vi "BLACK BOX FINDER.vi"() -> ()   [LabVIEW 2015]
uses:
  <vilib>/userdefined/High Color/IMAQdx.ctl
  <vilib>/vision/driver/NI_Vision_Acquisition_Software.lvlib
  <resource>/objmgr/imaqdx.rc
panel:
  out "Objects (real-world) (Object Tracking 1)":T1(array[cluster])
  out "Video Modes":string
  in  "Video Mode":dbl min=0.0 max=5.0 step=1.0
  in  "Camera":T2
  out "Y Resoloution":i32
  out "X Resoloution":i32
  in  "Stop 2":bool
  out "Image":T3(plugin-control)
  out "Image 2":T3(plugin-control)
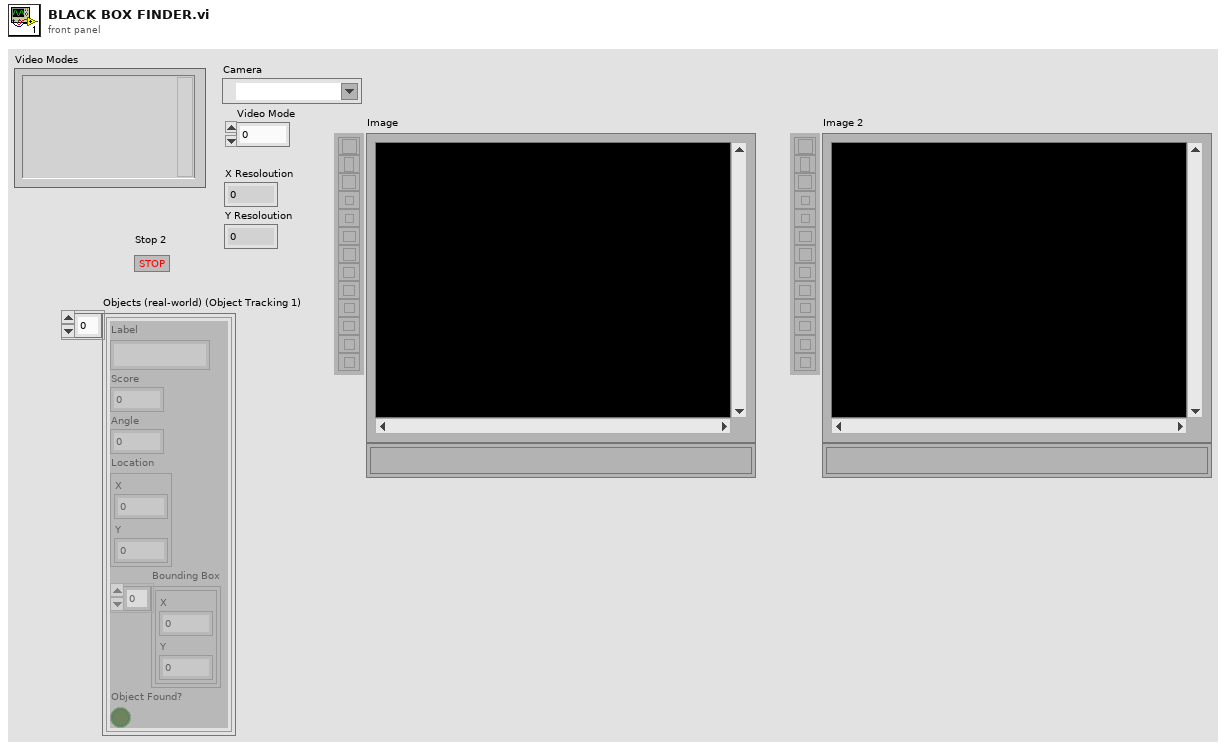
[diagram p1: front panel]
types:
  T1 = cluster{"Label":string, "Score":i32, "Angle":dbl, "Location":cluster{"X":dbl, "Y":dbl}, "Bounding Box":cluster{"X":dbl, "Y":dbl}[], "Object Found?":bool}[]
  T2 = typedef "IMAQdx.ctl" = refnum<k21>
  T3 = typedef "IMAQ Image.ctl" = refnum<image>
  T4 = typedef "IMAQ Point" = cluster{"X":sgl, "Y":sgl}
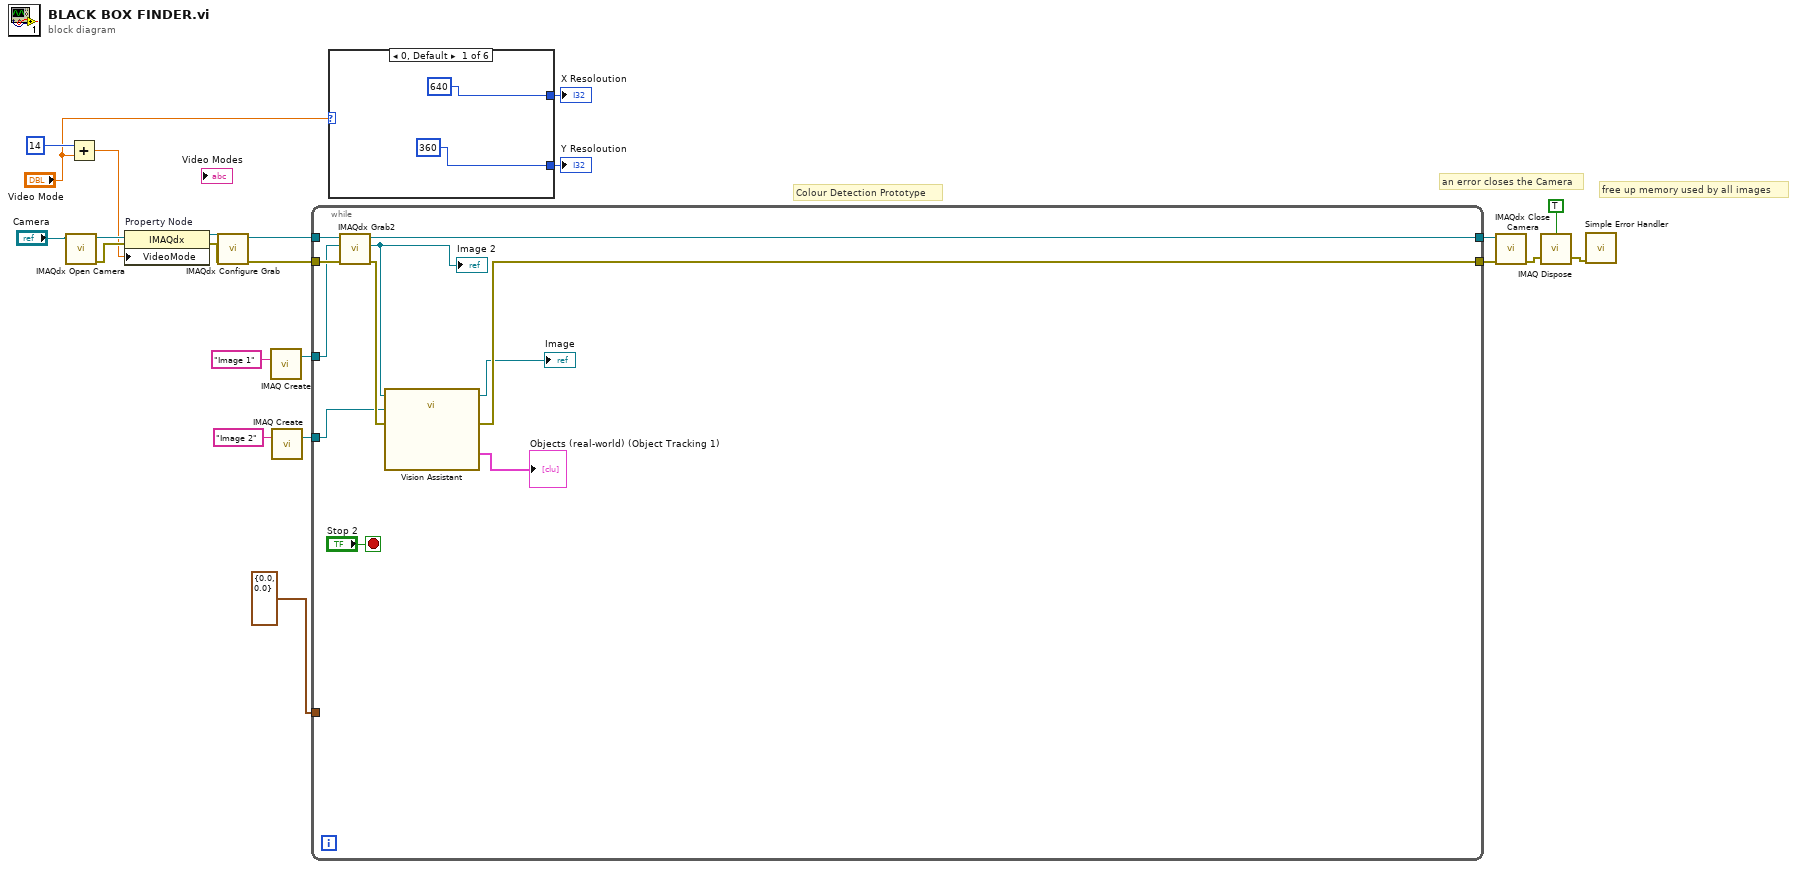
[diagram p0: block diagram]
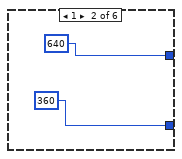
[diagram p2: hidden frame]
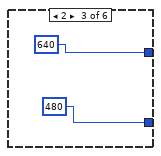
[diagram p3: hidden frame]
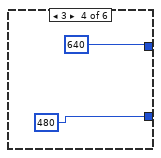
[diagram p4: hidden frame]
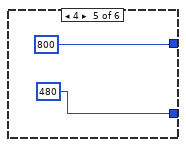
[diagram p5: hidden frame]
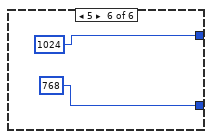
[diagram p6: hidden frame]
diagram:
  # "Colour Detection Prototype"
  # "an error closes the Camera"
  # "free up memory used by all images"
  n1 = call <vilib>:"IMAQdx Open Camera.vi"("Session In"="Camera") -> ("error out"=w12:errorcluster, "Session Out"=w13:T2)  [unwired: 9 in]
  n2 = Add(x=14, y="Video Mode") -> (x+y=w7:dbl)
  n3 = property on="Property Node" class="IMAQdx"(reference=w13, error in=w12, "VideoMode"=w7) -> (reference out=w11:T2, error out=w10:errorcluster)
  n4 = call <vilib>:"IMAQdx Configure Grab.vi"("error in"=w10, "Session In"=w11) -> ("error out"=w2:errorcluster, "Session Out"=w3:T2)  [unwired: 8 in]
  n5 = call "IMAQ Create"("Image Name"="Image 1") -> ("New Image"=w16:T3)  [unwired: 4 in, 1 out]
  n6 = call "IMAQ Create"("Image Name"="Image 2") -> ("New Image"=w19:T3)  [unwired: 4 in, 1 out]
  n7 = while {
    tunnel: [w26] -> w15
    tunnel: w19 -> [w24]
    tunnel: w2 -> [w33]
    tunnel: w3 -> [w32]
    tunnel: w16 -> [w31]
    tunnel: [w30] -> w14
    tunnel: T4 {"X"=0.0, "Y"=0.0} ("Point") -> [_]
    stop <- "Stop 2" stop-if-true
    n8 = call <vilib>:"IMAQdx Grab2.vi"("error in"=w33, "Image In"=w31, "Session In"=w32) -> ("error out"=w28:errorcluster, "Image Out"=w27:T3, "Session Out"=w30:T2)  [unwired: 5 in, 1 out]
    "Image 2" <- w27
    n9 = call "Vision Assistant"("Image In"=w27, "Image Dst"=w24, "error in"=w28) -> ("Image Out"=→"Image":T3, "Objects (real-world) (Object Tracking 1)"=→"Objects (real-world) (Object Tracking 1)":T1, "error out"=w26:errorcluster)  [unwired: 1 in, 21 out]
  }
  n10 = case shown="0, Default" "Video Mode" {
    tunnel: [640 640 640 640 800 1024] -> w4
    tunnel: [360 360 480 480 480 768] -> w5
    frame 0, Default {
    }
    frame 1 {
    }
    frame 2 {
    }
    frame 3 {
    }
    frame 4 {
    }
    frame 5 {
    }
  }
  "X Resoloution" <- w4
  "Y Resoloution" <- w5
  n11 = call <vilib>:"IMAQdx Close Camera.vi"("error in"=w15, "Session In"=w14) -> ("error out"=w20:errorcluster)  [unwired: 9 in]
  n12 = call "IMAQ Dispose"("All Images? (No)"=TRUE, "error in (no error)"=w20) -> ("error out"=w21:errorcluster)  [unwired: 4 in]
  n13 = call <vilib>:"Simple Error Handler.vi"("error in (no error)"=w21) -> ()  [unwired: 4 in, 5 out]
